vi "UMLEditor AddToolsMenuItems.vi"(0 "menu":refnum<k9>, 3 "GoopWizExists":bool, 5 "error in (no error)":errorcluster) -> (19 "error out":errorcluster)   [LabVIEW 2012]
doc: "Gets current diagram values"
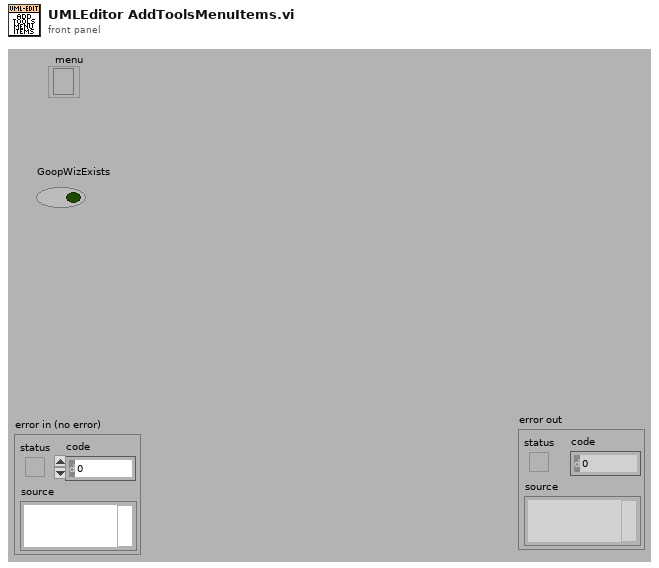
[diagram p1: front panel]
types:
  T1 = cluster{string, string, "short cut":cluster{"include Shift key?":bool, "shortcut key":string}}[]
  T2 = cluster{string, string, "short cut":cluster{"include Shift key?":bool, "shortcut key":string}}
  T3 = cluster{"include Shift key?":bool, "shortcut key":string}
  T4 = cluster{"include Shift key?":bool, "include Ctrl key? ":bool, "shortcut key":string}
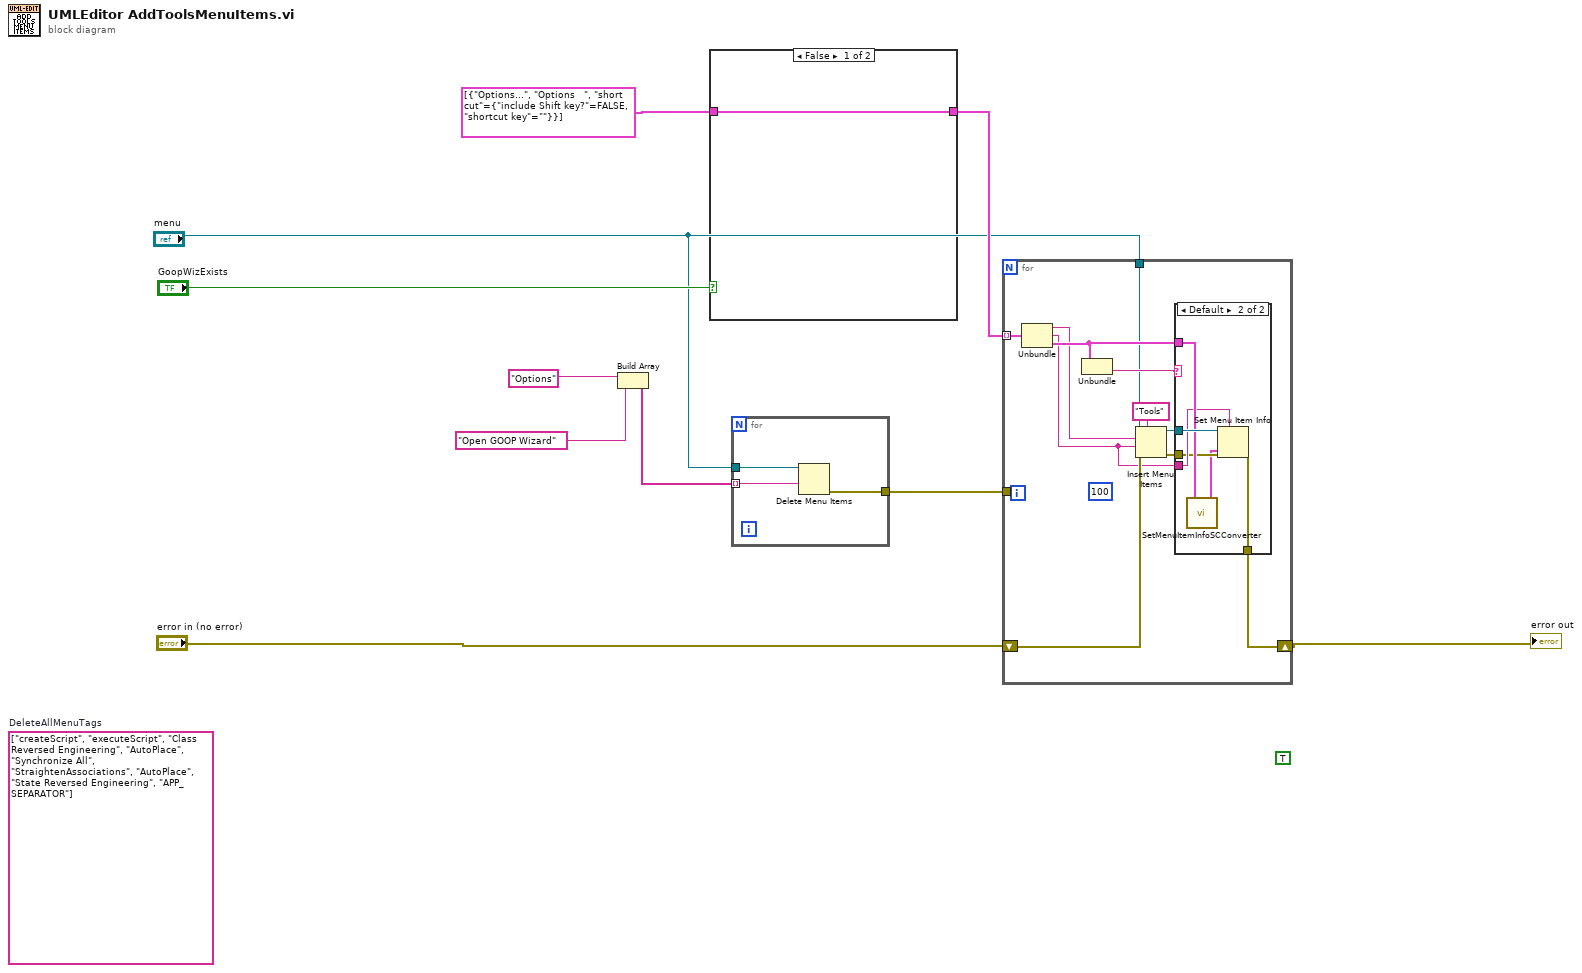
[diagram p0: block diagram]
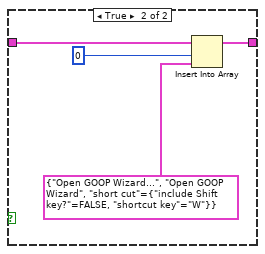
[diagram p2: hidden frame]
diagram:
  (unwired) TRUE
  (unwired) string[] ["createScript", "executeScript", "Class Reversed Engineering", "AutoPlace", "Synchronize All", "StraightenAssociations", "AutoPlace", "State Reversed Engineering", "APP_SEPARATOR"]  # DeleteAllMenuTags
  n1 = Build Array("Options", "Open GOOP Wizard") -> (w1:string[])
  n2 = case shown="False" "GoopWizExists" {
    tunnel: [w11 w15] -> w8
    tunnel: T1 [{"Options...", "Options   ", "short cut"={"include Shift key?"=FALSE, "shortcut key"=""}}] -> [w11 w12]
    frame False {
    }
    frame True {
      n3 = Insert Into Array(array=w12, index=0, new element=T2 {"Open GOOP Wizard...", "Open GOOP Wizard", "short cut"={"include Shift key?"=FALSE, "shortcut key"="W"}}) -> (w15:T1)
    }
  }
  n4 = for {
    tunnel: [w18] -> w5
    tunnel: "menu" -> [w17]
    tunnel: w1 -> [w16] mode=indexing
    n5 = Delete Menu Items(7:w16, 9:w17) -> (0:w18:errorcluster)  [unwired: 1 in, 2 out]
  }
  n6 = for {
    tunnel: w8 -> [w27] mode=indexing
    shift-right: [w20] -> w9
    shift-left: "error in (no error)" -> [w26]
    tunnel: "menu" -> [w21]
    tunnel: w5 -> [_]
    (unwired) 100
    n7 = Unbundle(w27) -> (w24:string, w23:string, "short cut"=w25:T3)
    n8 = Unbundle(w25) -> ("shortcut key"=w22:string)  [unwired: 1 out]
    n9 = Insert Menu Items(5:"Tools" ("menu tag"), 6:w26, 7:w23, 8:w24, 9:w21) -> (0:w19:errorcluster, 3:w28:refnum<k9>)  [unwired: 2 out]
    n10 = case shown="Default" w22 {
      tunnel: w28 -> [_ w36]
      tunnel: w25 -> [_ w35]
      tunnel: w23 -> [_ w34]
      tunnel: [w30 w33] -> w20
      tunnel: w19 -> [w30 w32]
      frame "" {
      }
      frame Default {
        n11 = call <vilib>:"SetMenuItemInfoSCConverter.vi"("short cut in"=w35) -> ("short cut out"=w31:T4)
        n12 = Set Menu Item Info(4:w31, 7:w34, 8:w32, 11:w36) -> (0:w33:errorcluster)  [unwired: 4 out]
      }
    }
  }
  "error out" <- w9
